vi "mainActivity_加载应用信息.vi"(11 "簇":T1) -> (0 "错误输出":errorcluster)   [LabVIEW 2014]
uses:
  R/manifest.vi
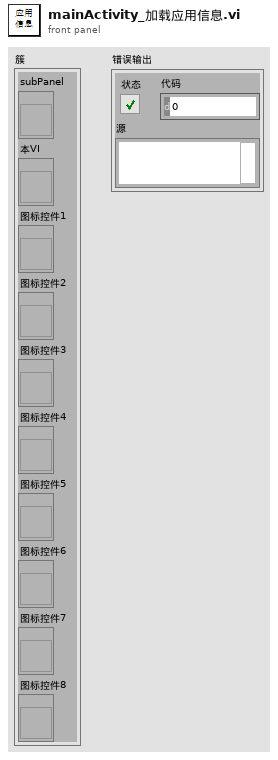
[diagram p1: front panel]
types:
  T1 = cluster{"subPanel":refnum<vi>, "本VI":refnum<vi>, "图标控件1":refnum<vi>, "图标控件2":refnum<vi>, "图标控件3":refnum<vi>, "图标控件4":refnum<vi>, "图标控件5":refnum<vi>, "图标控件6":refnum<vi>, "图标控件7":refnum<vi>, "图标控件8":refnum<vi>}
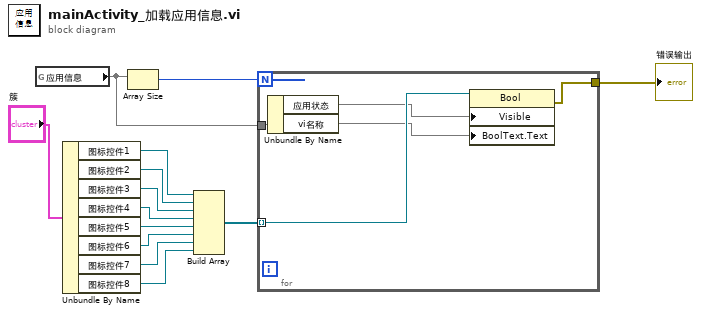
[diagram p0: block diagram]
diagram:
  n1 = global read "manifest.vi" "应用信息"() -> (w13)
  n2 = Unbundle By Name("簇") -> ("图标控件1"=w2:refnum<vi>, "图标控件2"=w3:refnum<vi>, "图标控件3"=w4:refnum<vi>, "图标控件4"=w5:refnum<vi>, "图标控件5"=w6:refnum<vi>, "图标控件6"=w7:refnum<vi>, "图标控件7"=w8:refnum<vi>, "图标控件8"=w9:refnum<vi>)
  n3 = Array Size(array=w13) -> (size(s)=w11:i32)
  n4 = Build Array(w2, w3, w4, w5, w6, w7, w8, w9) -> (w10:refnum<vi>[])
  n5 = for {
    N: w11 -> [_]
    tunnel: w10 -> [w18] mode=indexing
    tunnel: w13 -> [w17]
    tunnel: [w15] -> w12
    n6 = Unbundle By Name(w17) -> ("应用状态"=w14, "vi名称"=w16)
    n7 = property class="Bool"(reference=w18, "Visible"=w14, "BoolText.Text"=w16) -> (error out=w15:errorcluster)  [unwired: 1 in, 1 out]
  }
  "错误输出" <- w12
